vi "udp_receiver_sample.vi"() -> ()   [LabVIEW 2025]
panel:
  in  "Boolean 2":bool
  out "Waveform Graph":dbl[](graph)
  in  "Boolean":bool
  out "error out":errorcluster
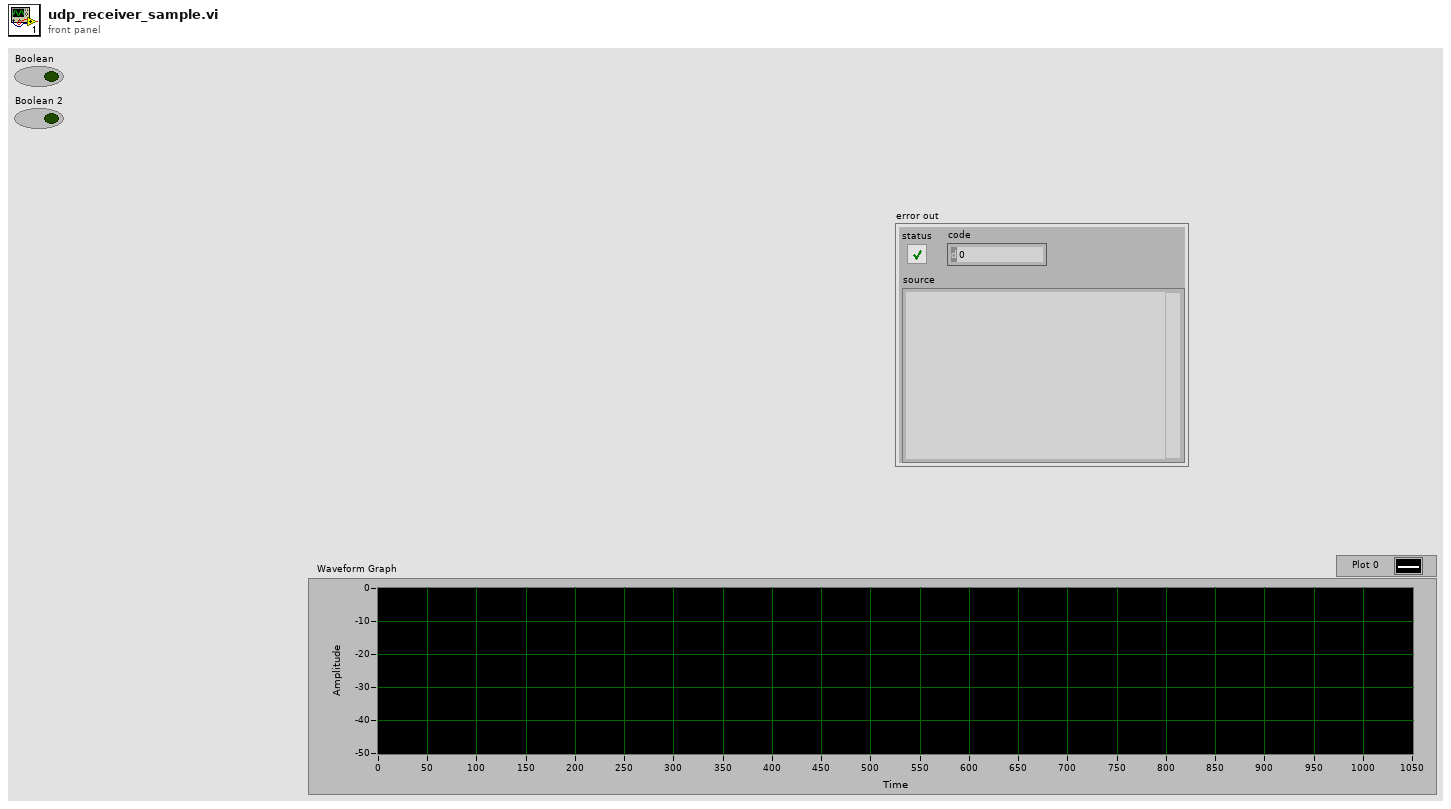
[diagram p1: front panel]
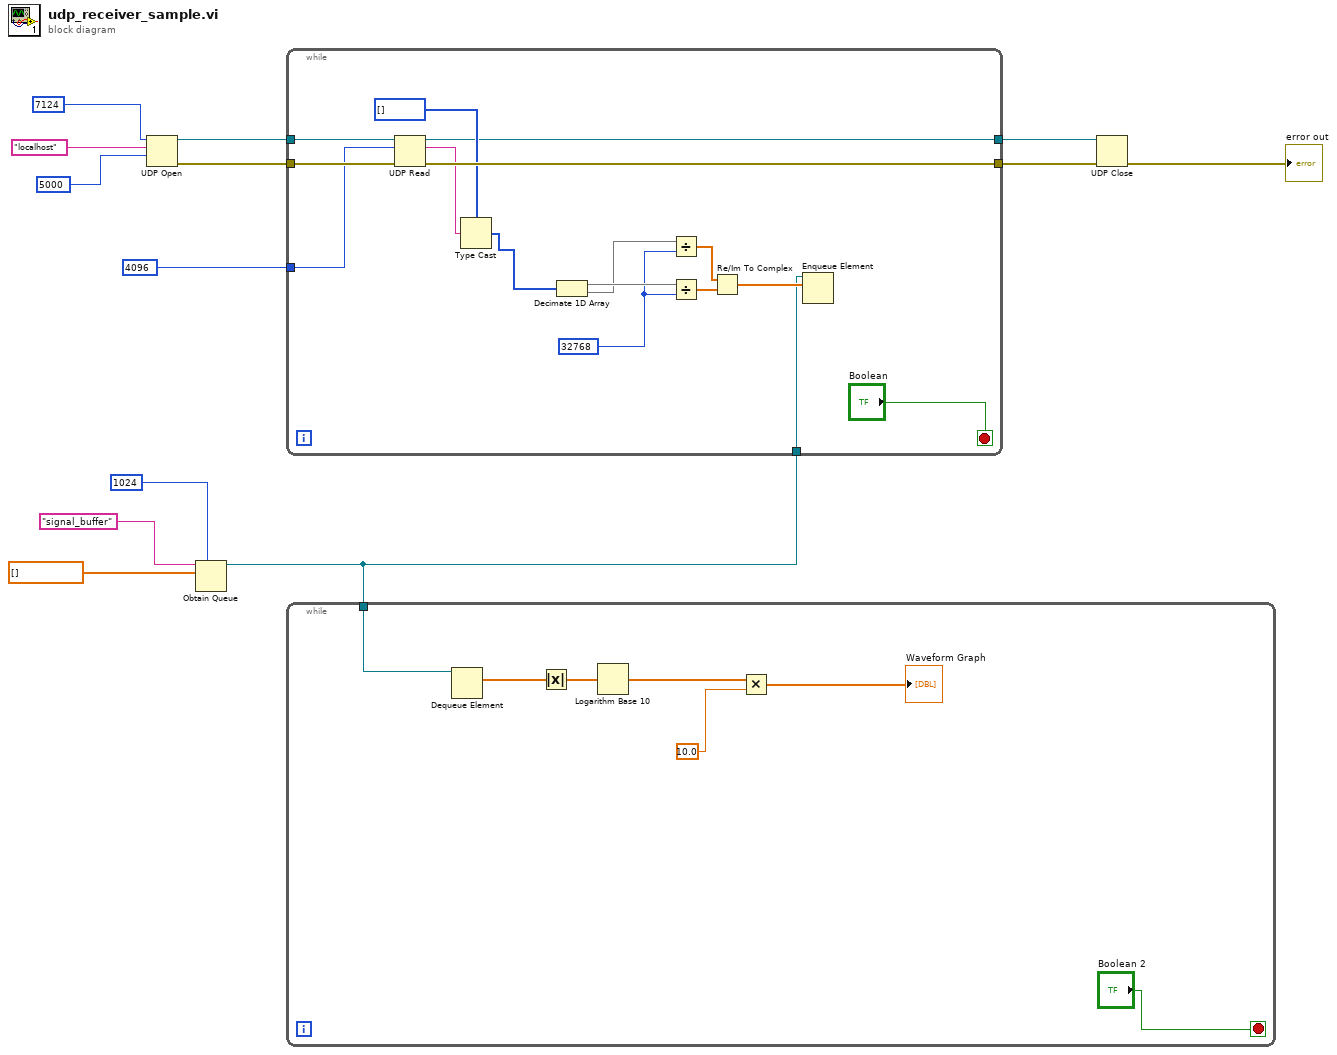
[diagram p0: block diagram]
diagram:
  n1 = UDP Open(9:5000 ("timeout ms (25000)"), 10:"localhost" ("service name"), 11:u16 7124 ("port")) -> (port=w13:refnum<k16>, 0:w9:errorcluster)  [unwired: 2 in, 1 out]
  n2 = Obtain Queue(max queue size (-1, unlimited)=1024, name (unnamed)="signal_buffer", element data type=cdb[] [] ("x + iy")) -> (queue out=w1:refnum<queue>)  [unwired: 2 in, 2 out]
  n3 = while {
    tunnel: w13 -> [w29]
    tunnel: w9 -> [w28]
    tunnel: [w27] -> w8
    tunnel: [w24] -> w7
    tunnel: 4096 ("max size (548)") -> [w22]
    tunnel: w1 -> [w14]
    stop <- "Boolean" stop-if-true
    w17 = 32768 ("FFT size")
    n4 = UDP Read(connection ID=w29, max size (548)=w22, 8:w28) -> (data out=w23:string, error out=w27:errorcluster, 3:w24:refnum<k16>)  [unwired: 1 in, 2 out]
    n5 = Type Cast(type=i16[] [] ("array"), x=w23) -> (*(type *) &x=w21:i16[])
    n6 = Decimate 1D Array(w21) -> (w20:i16[], w18:i16[])
    n7 = Divide(x=w18, y=w17) -> (x/y=w16:dbl[])
    n8 = Divide(x=w20, y=w17) -> (x/y=w19:dbl[])
    n9 = Re/Im To Complex(1:w19, 2:w16) -> (0:w15:cdb[])
    n10 = Enqueue Element(queue=w14, element=w15) -> ()  [unwired: 2 in, 3 out]
  }
  n11 = while {
    tunnel: w1 -> [w36]
    stop <- "Boolean 2" stop-if-true
    n12 = Dequeue Element(queue=w36) -> (element=w35:cdb[])  [unwired: 2 in, 3 out]
    n13 = Absolute Value(x=w35) -> (abs(x)=w34:dbl[])
    n14 = Logarithm Base 10(1:w34) -> (0:w33:dbl[])
    n15 = Multiply(x=w33, y=10.0) -> (x*y=→"Waveform Graph":dbl[])
  }
  n16 = UDP Close(connection ID=w7, 8:w8) -> (error out=→"error out":errorcluster)  [unwired: 1 out]
